vi "FPGA Target 2.vi"() -> ()   [LabVIEW 2015]
uses:
  <vilib>/Platform/TimedLoop/XDataNode/wakeup.ctl
  <vilib>/Platform/TimedLoop/XDataNode/XDNodeRunTimeDep.lvlib
  <vilib>/Platform/TimedLoop/XDataNode/nitl_modes.ctl
  <vilib>/Platform/TimedLoop/XDataNode/timing_clust.ctl
  <vilib>/Platform/TimedLoop/XDataNode/XDataNode.xnode
  <vilib>/NI/Engine Simulation Toolkit (EST)/APU/APU.lvlib
  <vilib>/rvi/DataTransferAndStorage/Container/XNode/niFpgaContainer.xnode
  <vilib>/rvi/interface/RandomDataEmulation/nirviRandomDataFpgaReadWriteTemplate.vi
  <vilib>/NI/Engine Simulation Toolkit (EST)/Digital Pattern Generation/Digital Pattern Generation.lvlib
  <vilib>/NI/Engine Simulation Toolkit (EST)/Directional Speed/Directional Speed.lvlib
  <vilib>/NI/Engine Simulation Toolkit (EST)/Analog Replay/Analog Replay.lvlib
  <vilib>/NI/FPGA Addon IP/Speciality IO/Speciality FPGA IO.lvlib
  <vilib>/NI/Engine Simulation Toolkit (EST)/Knock Sensor/Knock Sensor.lvlib
  <vilib>/NI/Engine Simulation Toolkit (EST)/ECU Event/Timing/ECU Event Timing.lvlib
  <vilib>/NI/Engine Simulation Toolkit (EST)/ECU Event/Timing/Measure Events (Non-40MHz).vi
  <vilib>/NI/Engine Simulation Toolkit (EST)/ECU Event/Timing/Capture Settings.ctl
  <vilib>/NI/Engine Simulation Toolkit (EST)/APU/Shared Settings.ctl
  <vilib>/NI/Engine Simulation Toolkit (EST)/Version Token.ctl
  <vilib>/NI/Engine Simulation Toolkit (EST)/Engine Simulation Toolkit.lvlib
  <vilib>/NI/Engine Simulation Toolkit (EST)/APU/Settings.ctl
  <vilib>/NI/Engine Simulation Toolkit (EST)/APU/Input.ctl
  <vilib>/NI/Engine Simulation Toolkit (EST)/APU/Output.ctl
  <vilib>/NI/Engine Simulation Toolkit (EST)/Digital Pattern Generation/Load Input.ctl
  <vilib>/NI/Engine Simulation Toolkit (EST)/Directional Speed/Load Input.ctl
  <vilib>/NI/Engine Simulation Toolkit (EST)/Analog Replay/Load Input.ctl
  <vilib>/NI/FPGA Addon IP/Speciality IO/Types/PWM.Measure.Analog.Settings.ctl
  <vilib>/NI/FPGA Addon IP/Speciality IO/Types/PWM.Measure.Analog.Measurement.ctl
  <vilib>/NI/Engine Simulation Toolkit (EST)/Knock Sensor/Cylinder Settings.ctl
  <vilib>/NI/Engine Simulation Toolkit (EST)/Knock Sensor/Cylinder Input.ctl
  <vilib>/NI/Engine Simulation Toolkit (EST)/Knock Sensor/Generate Settings.ctl
  <vilib>/NI/Engine Simulation Toolkit (EST)/Knock Sensor/Generate Input.ctl
  <vilib>/NI/Engine Simulation Toolkit (EST)/Analog Replay/Input.ctl
  <vilib>/NI/Engine Simulation Toolkit (EST)/Analog Replay/Settings.ctl
  <vilib>/NI/FPGA Addon IP/Speciality IO/Types/Sine.Generate.Settings.ctl
  <vilib>/NI/FPGA Addon IP/Speciality IO/Types/PWM.Generate.Digital.Settings.ctl
  <vilib>/NI/Engine Simulation Toolkit (EST)/Digital Pattern Generation/Input.ctl
  <vilib>/NI/Engine Simulation Toolkit (EST)/Digital Pattern Generation/Settings.ctl
  <vilib>/NI/Engine Simulation Toolkit (EST)/Directional Speed/Input.ctl
  <vilib>/NI/Engine Simulation Toolkit (EST)/Directional Speed/Settings.ctl
  <vilib>/NI/FPGA Addon IP/Speciality IO/Types/WSS.Generate.Digital.Settings.ctl
  <vilib>/NI/FPGA Addon IP/Speciality IO/Types/PWM.Measure.Digital.Settings.ctl
  <vilib>/NI/FPGA Addon IP/Speciality IO/Types/PWM.Measure.Digital.Measurement.ctl
  <vilib>/NI/Engine Simulation Toolkit (EST)/ECU Event/Timing/Measure Settings.ctl
  <vilib>/NI/Engine Simulation Toolkit (EST)/ECU Event/Timing/Measure Output.ctl
  <vilib>/NI/Engine Simulation Toolkit (EST)/ECU Event/Timing/Capture Output.ctl
panel:
  out "capture.Cyl Inj 3.Event 4":T1
  out "capture.Cyl Inj 3.Event 3":T1
  out "capture.Cyl Inj 3.Event 2":T1
  out "capture.Cyl Inj 3.Event 1":T1
  out "status.Cyl Inj 3":T2
  in  "settings.Cyl Inj 3":T3
  out "capture.Cyl Inj 2.Event 4":T1
  out "capture.Cyl Inj 2.Event 3":T1
  out "capture.Cyl Inj 2.Event 2":T1
  out "capture.Cyl Inj 2.Event 1":T1
  out "status.Cyl Inj 2":T2
  in  "settings.Cyl Inj 2":T3
  out "capture.Cyl Inj 1.Event 4":T1
  out "capture.Cyl Inj 1.Event 3":T1
  out "capture.Cyl Inj 1.Event 2":T1
  out "capture.Cyl Inj 1.Event 1":T1
  out "status.Cyl Inj 1":T2
  in  "settings.Cyl Inj 1":T3
  out "PWM IN 2.Measure":T4
  in  "PWM IN 2.Settings":T5={"ACTIVE EDGE"=TRUE, "TIMEOUT"=40000000}
  out "PWM IN 1.Measure":T4
  in  "PWM IN 1.Settings":T5={"ACTIVE EDGE"=TRUE, "TIMEOUT"=40000000}
  out "Key State":bool
  out "Switch State":bool
  out "Relay State":bool
  out "Connector0 DIO Bank2.Monitor":bool[](array[boolean])
  out "Connector0 DIO Bank1.Monitor":bool[](array[boolean])
  in  "Read Passenger WS.Settings":T6={"ACTIVE EDGE"=TRUE, "ACTIVE TICKS"=0, "INACTIVE TICKS"=0, "DATA"=0, "SENSOR TYPE"=0}
  in  "Rear Driver WS.Settings":T6={"ACTIVE EDGE"=TRUE, "ACTIVE TICKS"=0, "INACTIVE TICKS"=0, "DATA"=0, "SENSOR TYPE"=0}
  in  "Front Passenger WS.Settings":T6={"ACTIVE EDGE"=TRUE, "ACTIVE TICKS"=0, "INACTIVE TICKS"=0, "DATA"=0, "SENSOR TYPE"=0}
  in  "Front Driver WS.Settings":T6={"ACTIVE EDGE"=TRUE, "ACTIVE TICKS"=0, "INACTIVE TICKS"=0, "DATA"=0, "SENSOR TYPE"=0}
  out "Connector0 DIO Bank0.Monitor":bool[](array[boolean])
  in  "input.Crank":T7
  in  "settings.Crank":T8
  in  "input.Crank_Temp":T9
  in  "settings.Crank_Temp":T10
  in  "Switch":bool
  in  "Key":bool
  in  "input.Exhaust CAM 1":T9
  in  "settings.Exhaust CAM 1":T10
  in  "input.Intake CAM 1":T9
  in  "settings.Intake CAM 1":T10
  in  "PWM Out 2.Settings":T11={"ACTIVE EDGE"=TRUE, "ACTIVE TICKS"=0, "INACTIVE TICKS"=0}
  in  "PWM Out 1.Settings":T11={"ACTIVE EDGE"=TRUE, "ACTIVE TICKS"=0, "INACTIVE TICKS"=0}
  out "Connector1 AO Bank0.Monitor":fxp<+/-,32,8>[](array[numeric])
  in  "Simple Knock 2.Settings":T12={"AMP"=0.0, "OFFSET"=0.0, "PERIODS/TICKS"=2.4999957531690598e-05}
  in  "Simple Knock 1.Settings":T12={"AMP"=0.0, "OFFSET"=0.0, "PERIODS/TICKS"=2.4999957531690598e-05}
  in  "input.VR Sensor2":T13
  in  "settings.VR Sensor2":T14
  in  "input.VR Sensor1":T13
  in  "settings.VR Sensor1":T14
  in  "Power Supply Setpoint":fxp<+/-,32,8> format="%#_27g"
  in  "Dyno Setpoint":fxp<+/-,32,8> format="%#_27g"
  in  "input.Knock2":T15
  in  "settings.Knock2":T16
  in  "input.Knock2.Cylinder 7":T17={"probability compare"=65535, "high freq scaler"=0.0, "trigger position"=0}
  in  "settings.Knock2.Cylinder 7":T18
  in  "input.Knock2.Cylinder 6":T17={"probability compare"=65535, "high freq scaler"=0.0, "trigger position"=0}
  in  "settings.Knock2.Cylinder 6":T18
  in  "input.Knock2.Cylinder 5":T17={"probability compare"=65535, "high freq scaler"=0.0, "trigger position"=0}
  in  "settings.Knock2.Cylinder 5":T18
  in  "input.Knock2.Cylinder 4":T17={"probability compare"=65535, "high freq scaler"=0.0, "trigger position"=0}
  in  "settings.Knock2.Cylinder 4":T18
  in  "input.Knock2.Cylinder 3":T17={"probability compare"=65535, "high freq scaler"=0.0, "trigger position"=0}
  in  "settings.Knock2.Cylinder 3":T18
  in  "input.Knock2.Cylinder 2":T17={"probability compare"=65535, "high freq scaler"=0.0, "trigger position"=0}
  in  "settings.Knock2.Cylinder 2":T18
  in  "input.Knock2.Cylinder 1":T17={"probability compare"=65535, "high freq scaler"=0.0, "trigger position"=0}
  in  "settings.Knock2.Cylinder 1":T18
  in  "input.Knock1":T15
  in  "settings.Knock1":T16
  in  "input.Knock1.Cylinder 6":T17={"probability compare"=65535, "high freq scaler"=0.0, "trigger position"=0}
  in  "settings.Knock1.Cylinder 6":T18
  in  "input.Knock1.Cylinder 5":T17={"probability compare"=65535, "high freq scaler"=0.0, "trigger position"=0}
  in  "settings.Knock1.Cylinder 5":T18
  in  "input.Knock1.Cylinder 4":T17={"probability compare"=65535, "high freq scaler"=0.0, "trigger position"=0}
  in  "settings.Knock1.Cylinder 4":T18
  in  "input.Knock1.Cylinder 3":T17={"probability compare"=65535, "high freq scaler"=0.0, "trigger position"=0}
  in  "settings.Knock1.Cylinder 3":T18
  in  "input.Knock1.Cylinder 2":T17={"probability compare"=65535, "high freq scaler"=0.0, "trigger position"=0}
  in  "settings.Knock1.Cylinder 2":T18
  in  "input.Knock1.Cylinder 1":T17={"probability compare"=65535, "high freq scaler"=0.0, "trigger position"=0}
  in  "settings.Knock1.Cylinder 1":T18
  out "Temp2":fxp<+/-,32,8> format="%#_27g"
  out "Temp1":fxp<+/-,32,8> format="%#_27g"
  out "Pressure4":fxp<+/-,32,8> format="%#_27g"
  out "Pressure3":fxp<+/-,32,8> format="%#_27g"
  out "Injector4.Measure":T19
  in  "Injector4.Settings":T20={"ACTIVE EDGE"=TRUE, "TIMEOUT"=40000000, "THRESHOLD"=50.0}
  out "Injector3.Measure":T19
  in  "Injector3.Settings":T20={"ACTIVE EDGE"=TRUE, "TIMEOUT"=40000000, "THRESHOLD"=50.0}
  out "Pressure2":fxp<+/-,32,8> format="%#_27g"
  out "Pressure1":fxp<+/-,32,8> format="%#_27g"
  out "Connector1 AI Bank0.Monitor":fxp<+/-,27,5>[](array[numeric])
  in  "load input.VR Sensor2":T21={"Data"=[0, 0, 0, 0, 0, 0, 0, 0, 0, 0, 0, 0, 0, 0, 0, 0], "LoadOffset"=0, "Done"=FALSE}
  in  "load input.VR Sensor1":T21={"Data"=[0, 0, 0, 0, 0, 0, 0, 0, 0, 0, 0, 0, 0, 0, 0, 0], "LoadOffset"=0, "Done"=FALSE}
  in  "load input.Crank":T22
  in  "load input.Crank_Temp":T23
  in  "load input.Exhaust CAM 1":T23
  in  "load input.Intake CAM 1":T23
  in  "Analog Input Loop Timer (uSec)":u32
  out "output.apu 1":T24 caption="output"
  in  "input.apu 1":T25={"desired speed"=0.0, "reset"=TRUE} caption="input"
  in  "settings.apu 1":T26 caption="settings"
  in  "est.version":T27
  in  "shared settings.apu 1":T28 {"start" format="%#.15g"}
  in  "go.apu 1":bool
  in  "Digital Loop Timer (uSec)":u32
  in  "Analog Output Loop Timer (uSec)":u32
  in  "DMA.Enable":bool
  in  "DMA.MinimumSamples":u32 caption="DMA Loop Timer (uSec)"
  out "DMA.Timeout":bool
  in  "DMA.Timeout.Reset":bool
  in  "DMA Loop Timer (uSec)":u32
types:
  T1 = typedef "Engine Simulation Toolkit.lvlib/ECU Event Timing.lvlib/Capture Output.ctl" = cluster{"Start":u16, "End":u16, "Duration (tics)":fxp<+,18,18>, "Event present":bool}
  T2 = typedef "Engine Simulation Toolkit.lvlib/ECU Event Timing.lvlib/Measure Output.ctl" = cluster{"stuck active":bool, "window all active":bool, "window orphan start":bool, "window orphan end":bool}
  T3 = typedef "Engine Simulation Toolkit.lvlib/ECU Event Timing.lvlib/Measure Settings.ctl" = cluster{"max":u16, "min":u16, "active high":bool, "wrap":bool}
  T4 = typedef "Speciality FPGA IO.lvlib/PWM.Measure.Digital.Measurement.ctl" = cluster{"ACTIVE TICKS":u32, "INACTIVE TICKS":u32, "ACQ TICKS":u32}
  T5 = typedef "Speciality FPGA IO.lvlib/PWM.Measure.Digital.Settings.ctl" = cluster{"ACTIVE EDGE":bool, "TIMEOUT":u32}
  T6 = typedef "Speciality FPGA IO.lvlib/WSS.Generate.Digital.Settings.ctl" = cluster{"ACTIVE EDGE":bool, "ACTIVE TICKS":u32, "INACTIVE TICKS":u32, "DATA":u8, "SENSOR TYPE":u8}
  T7 = typedef "Engine Simulation Toolkit.lvlib/Directional Speed.lvlib/Settings.ctl" = cluster{"Upper Value":u16, "Lower Value":u16, "Upper Index":fxp<+,10,10>, "Lower Index":fxp<+,10,10>, "Enabled":bool}
  T8 = typedef "Engine Simulation Toolkit.lvlib/Directional Speed.lvlib/Input.ctl" = cluster{"td (tics)":u16, "tf (tics)":u16, "tr (tics)":u16}
  T9 = typedef "Engine Simulation Toolkit.lvlib/Digital Pattern Generation.lvlib/Settings.ctl" = cluster{"edge 1":u16, "edge 2":u16, "cycle angle":bool, "enabled":bool, "first falling":bool, "fault":bool, "fault wrap":bool, "fault value":bool, "fault count":fxp<+,4,4>, "use fault count":bool}
  T10 = typedef "Engine Simulation Toolkit.lvlib/Digital Pattern Generation.lvlib/Input.ctl" = cluster{"Offset":i16}
  T11 = typedef "Speciality FPGA IO.lvlib/PWM.Generate.Digital.Settings.ctl" = cluster{"ACTIVE EDGE":bool, "ACTIVE TICKS":u32, "INACTIVE TICKS":u32}
  T12 = typedef "Speciality FPGA IO.lvlib/Sine.Generate.Settings.ctl" = cluster{"AMP":fxp<+/-,32,8>, "OFFSET":fxp<+/-,32,8>, "PERIODS/TICKS":fxp<+,32,0>}
  T13 = typedef "Engine Simulation Toolkit.lvlib/Analog Replay.lvlib/Settings.ctl" = cluster{"ReverseNegate":bool, "CycleAngle":bool, "SpeedThreshold":fxp<+/-,23,2>, "AOBelowThreshold":i16}
  T14 = typedef "Engine Simulation Toolkit.lvlib/Analog Replay.lvlib/Input.ctl" = cluster{"Offset":i16, "VScaleSlope":fxp<+,18,6>, "VScaleIntercept":fxp<+/-,18,3>}
  T15 = typedef "Engine Simulation Toolkit.lvlib/Knock Sensor.lvlib/Generate Input.ctl" = cluster{"low freq scaler":fxp<+,10,0>}
  T16 = typedef "Engine Simulation Toolkit.lvlib/Knock Sensor.lvlib/Generate Settings.ctl" = cluster{"low freq (periods/tick)":fxp<+,32,0>, "high freq (periods/tick)":fxp<+,32,0>, "duration (1.25MHz tics)":fxp<+,18,18>, "low freq speed slope":fxp<+,16,-3>, "low freq speed intercept":fxp<+,10,-10>, "low freq by speed":bool}
  T17 = typedef "Engine Simulation Toolkit.lvlib/Knock Sensor.lvlib/Cylinder Input.ctl" = cluster{"probability compare":u16, "high freq scaler":fxp<+,10,0>, "trigger position":u16}
  T18 = typedef "Engine Simulation Toolkit.lvlib/Knock Sensor.lvlib/Cylinder Settings.ctl" = cluster{"seed":u16, "reset":bool}
  T19 = typedef "Speciality FPGA IO.lvlib/PWM.Measure.Analog.Measurement.ctl" = cluster{"ACTIVE TICKS":u32, "INACTIVE TICKS":u32, "ACQ TICKS":u32, "ACTIVE VOLTAGE":fxp<+/-,32,8>, "INACTIVE VOLTAGE":fxp<+/-,32,8>}
  T20 = typedef "Speciality FPGA IO.lvlib/PWM.Measure.Analog.Settings.ctl" = cluster{"ACTIVE EDGE":bool, "TIMEOUT":u32, "THRESHOLD":fxp<+/-,32,8>}
  T21 = typedef "Engine Simulation Toolkit.lvlib/Analog Replay.lvlib/Load Input.ctl" = cluster{"Data":i16[], "LoadOffset":u16, "Done":bool}
  T22 = typedef "Engine Simulation Toolkit.lvlib/Directional Speed.lvlib/Load Input.ctl" = cluster{"address":fxp<+,10,10>, "done":bool, "angle":u16}
  T23 = typedef "Engine Simulation Toolkit.lvlib/Digital Pattern Generation.lvlib/Load Input.ctl" = cluster{"address":fxp<+,11,11>, "done":bool, "angle":u16}
  T24 = typedef "Engine Simulation Toolkit.lvlib/APU.lvlib/Output.ctl" = cluster{"crank":u16, "cycle":u16, "actual speed":fxp<+/-,23,2>}
  T25 = typedef "Engine Simulation Toolkit.lvlib/APU.lvlib/Input.ctl" = cluster{"desired speed":fxp<+/-,23,2>, "reset":bool}
  T26 = typedef "Engine Simulation Toolkit.lvlib/APU.lvlib/Settings.ctl" = cluster{"acceleration":fxp<+,18,-20>, "enable accel":bool}
  T27 = typedef "Engine Simulation Toolkit.lvlib/Version Token.ctl" = cluster{"1.3.0":bool}
  T28 = typedef "Engine Simulation Toolkit.lvlib/APU.lvlib/Shared Settings.ctl" = cluster{"start":fxp<+,17,17>, "stuck limit":fxp<+,18,18>}
  T29 = typedef "XDNodeRunTimeDep.lvlib/timing_clust.ctl" = cluster{"Expected End [f-1]":u64, "Actual End [f-1]":u64, "Finished Late? [f-1]":bool, "Expected End [i-1]":u64, "Actual End [i-1]":u64, "Finished Late? [i-1]":bool, "Expected Start [i]":u64, "Actual Start [i]":u64, "Expected Start [f]":u64, "Actual Start [f]":u64, "Source Name":string, "Structure Name":string, "Period":i64, "Deadline":i64, "Offset":i64, "Start":i64, "Priority":i32, "Timeout":i32, "Mode":T30, "Wakeup Reason":T31, "Error":errorcluster, "Source Type":string, "Secondary Source Type":string, "Global End Time":u64, "Global Start Time":u64, "Frame Duration":u64, "Iteration Duration":u64, "Assigned CPU":i32, "I/O Scan Engine Mode":u32}
  T30 = typedef "XDNodeRunTimeDep.lvlib/nitl_modes.ctl" = enum32{"No Change", "Process missed periods, maintain original phase", "Discard missed periods, maintain original phase", "Process missed periods, ignore original phase", "Discard missed periods, ignore original phase"}
  T31 = typedef "XDNodeRunTimeDep.lvlib/wakeup.ctl" = enum32{"Normal", "Aborted", "Asynchronous wakeup", "Timing source error", "Timed loop error", "Timeout"}
  T32 = typedef "Engine Simulation Toolkit.lvlib/ECU Event Timing.lvlib/Capture Settings.ctl" = u8
  T33 = cluster{"DI 0":refnum<k21>, "DI 1":refnum<k21>, "DI 2":refnum<k21>, "DI 3":refnum<k21>, "DI 4":refnum<k21>, "DI 5":refnum<k21>, "DI 6":refnum<k21>, "DI 7":refnum<k21>}
  T34 = cluster{"DO 0":refnum<k21>, "DO 1":refnum<k21>, "DO 2":refnum<k21>, "DO 3":refnum<k21>, "DO 4":refnum<k21>, "DO 5":refnum<k21>, "DO 6":refnum<k21>, "DO 7":refnum<k21>}
  T35 = cluster{"AO 0":refnum<k21>, "AO 1":refnum<k21>, "AO 2":refnum<k21>, "AO 3":refnum<k21>, "AO 4":refnum<k21>, "AO 5":refnum<k21>, "AO 6":refnum<k21>, "AO 7":refnum<k21>}
  T36 = cluster{"AI 0":refnum<k21>, "AI 1":refnum<k21>, "AI 2":refnum<k21>, "AI 3":refnum<k21>, "AI 4":refnum<k21>, "AI 5":refnum<k21>, "AI 6":refnum<k21>, "AI 7":refnum<k21>}
  T37 = typedef "Engine Simulation Toolkit.lvlib/APU.lvlib/Register Bus.ctl" = cluster{"Speed":refnum<k21>, "Crank Angle":refnum<k21>, "Cycle Angle":refnum<k21>, "Crank Count":refnum<k21>, "Cycle Count":refnum<k21>, "1.25 MHz Counter":refnum<k21>, "Crank Rollover":refnum<k21>, "Cycle Rollover":refnum<k21>, "shared settings":T28}
  T38 = typedef "Engine Simulation Toolkit.lvlib/Digital Pattern Generation.lvlib/Load Data.ctl" = cluster{"max address":fxp<+,11,11>, "memory":refnum<k21>}
  T39 = typedef "Engine Simulation Toolkit.lvlib/Directional Speed.lvlib/Load Data.ctl" = cluster{"max address":fxp<+,10,10>, "Memory":refnum<k21>}
  T40 = typedef "Engine Simulation Toolkit.lvlib/Knock Sensor.lvlib/Triggered Cylinder Data.ctl" = cluster{"trigger knock":bool, "high freq scaler":fxp<+,10,0>}
  T41 = typedef "Engine Simulation Toolkit.lvlib/ECU Event Timing.lvlib/Measured Data.ctl" = cluster{"start":u16, "end":u16, "duration (tics)":fxp<+,18,18>, "window end":bool, "window begin":bool, "pulse end":bool, "pulse #":u8}
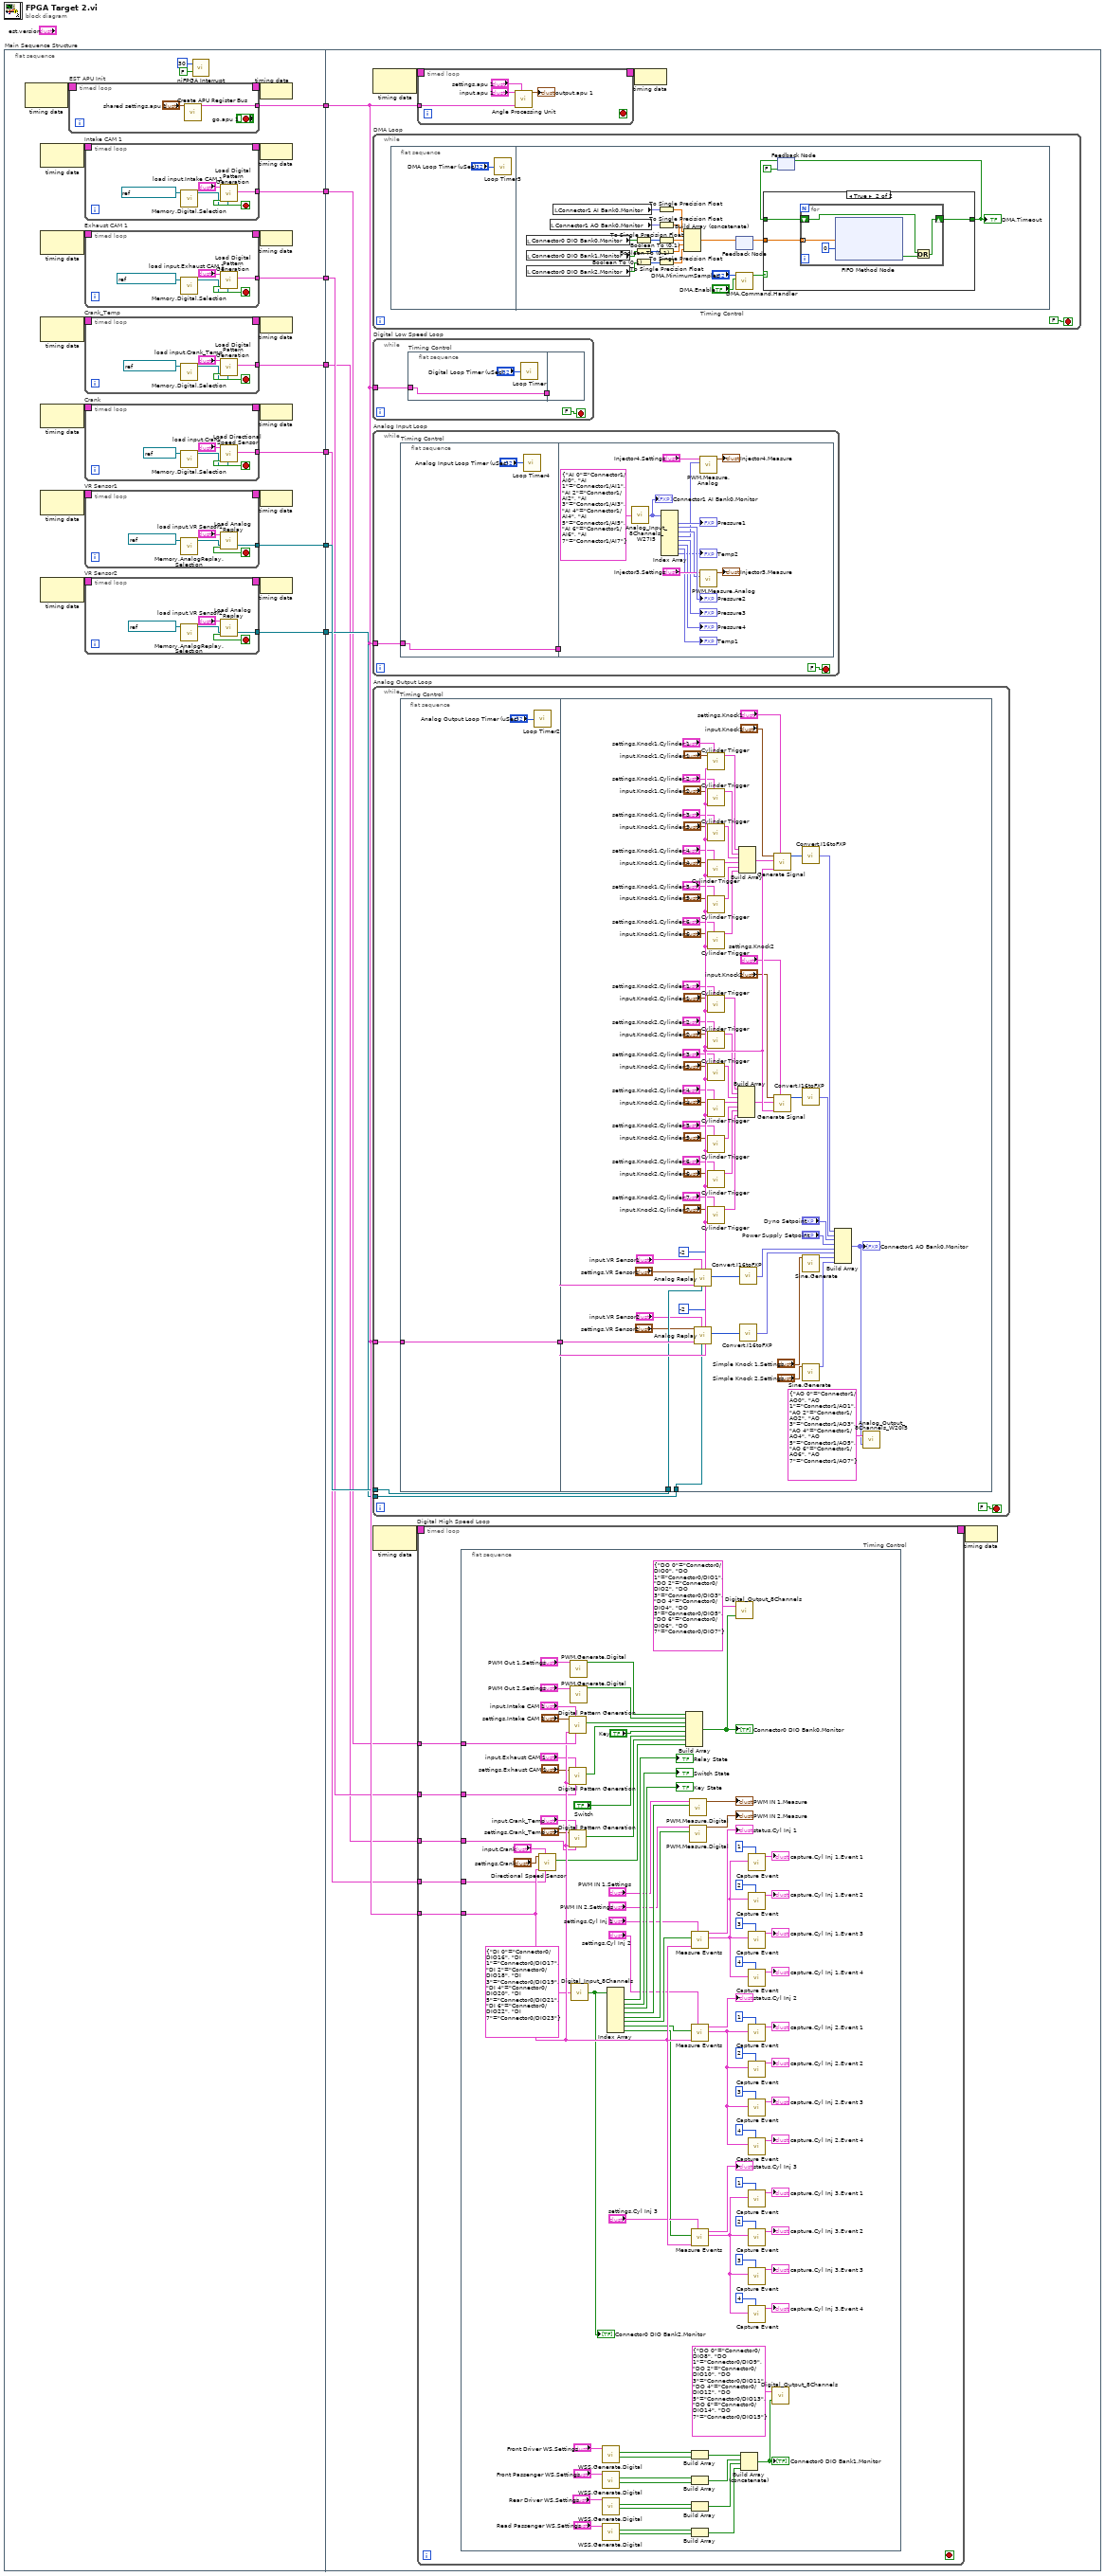
[diagram p0: block diagram]
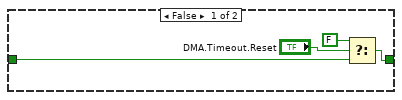
[diagram p2: hidden frame]
diagram:
  n1 = flat-sequence "Main Sequence Structure" {
    tunnel: [w26] -> w7
    tunnel: [w13] -> w6
    tunnel: [w12] -> w5
    tunnel: [w11] -> w4
    tunnel: [w10] -> w3
    tunnel: [w9] -> w2
    tunnel: [w8] -> w1
    tunnel: w7 -> [w96]
    tunnel: w6 -> [w95]
    tunnel: w5 -> [w94]
    tunnel: w4 -> [w93]
    tunnel: w3 -> [w92]
    tunnel: w2 -> [w91]
    tunnel: w1 -> [w90]
    frame #0 {
      n2 = node-c288() -> (w28:T29)  [unwired: 1 in]
      n3 = node-c288() -> (w25:T29)  [unwired: 1 in]
      n4 = node-c288() -> (w23:T29)  [unwired: 1 in]
      n5 = node-c288() -> (w21:T29)  [unwired: 1 in]
      n6 = node-c288() -> (w19:T29)  [unwired: 1 in]
      n7 = node-c288() -> (w17:T29)  [unwired: 1 in]
      n8 = node-c288() -> (w15:T29)  [unwired: 1 in]
      n9 = timed-loop "EST APU Init" {
        timing: w28 -> [_]
        timing-out: [_] -> w27
        tunnel: [w83] -> w26
        stop <- "go.apu 1" stop-if-true
        n10 = call <vilib>:"Create APU Register Bus.vi"("shared settings.<user name>"="shared settings.apu 1") -> ("register bus"=w83:T37)  [unwired: 10 in]
      }
      n11 = timed-loop "Intake CAM 1" {
        timing: w25 -> [_]
        timing-out: [_] -> w24
        tunnel: [w74] -> w11
        stop <- w77 stop-if-true
        n12 = call "Memory.Digital.Selection.vi"("memory"=refnum<k21> "Intake CAM 1") -> ("memory"=w75:refnum<k21>)  [unwired: 10 in]
        n13 = call <vilib>:"Load Digital Pattern Generation.vi"("memory"=w75, "load input.<user name>"="load input.Intake CAM 1") -> ("done"=w77:bool, "load data"=w74:T38)  [unwired: 8 in]
      }
      n14 = timed-loop "Exhaust CAM 1" {
        timing: w23 -> [_]
        timing-out: [_] -> w22
        tunnel: [w65] -> w10
        stop <- w68 stop-if-true
        n15 = call "Memory.Digital.Selection.vi"("memory"=refnum<k21> "Exhaust CAM 1") -> ("memory"=w66:refnum<k21>)  [unwired: 10 in]
        n16 = call <vilib>:"Load Digital Pattern Generation.vi"("memory"=w66, "load input.<user name>"="load input.Exhaust CAM 1") -> ("done"=w68:bool, "load data"=w65:T38)  [unwired: 8 in]
      }
      n17 = timed-loop "Crank_Temp" {
        timing: w21 -> [_]
        timing-out: [_] -> w20
        tunnel: [w56] -> w9
        stop <- w59 stop-if-true
        n18 = call "Memory.Digital.Selection.vi"("memory"=refnum<k21> "Crank_Temp") -> ("memory"=w57:refnum<k21>)  [unwired: 10 in]
        n19 = call <vilib>:"Load Digital Pattern Generation.vi"("memory"=w57, "load input.<user name>"="load input.Crank_Temp") -> ("done"=w59:bool, "load data"=w56:T38)  [unwired: 8 in]
      }
      n20 = timed-loop "Crank" {
        timing: w19 -> [_]
        timing-out: [_] -> w18
        tunnel: [w47] -> w8
        stop <- w50 stop-if-true
        n21 = call "Memory.Digital.Selection.vi"("memory"=refnum<k21> "Crank") -> ("memory"=w48:refnum<k21>)  [unwired: 10 in]
        n22 = call <vilib>:"Load Directional Speed Sensor.vi"("Memory In"=w48, "load input.<user name>"="load input.Crank") -> ("done"=w50:bool, "load data"=w47:T39)  [unwired: 8 in]
      }
      n23 = timed-loop "VR Sensor1" {
        timing: w17 -> [_]
        timing-out: [_] -> w16
        tunnel: [w39] -> w13
        stop <- w41 stop-if-true
        n24 = call "Memory.AnalogReplay.Selection.vi"("memory"=refnum<k21> "VR Sensor1") -> ("memory"=w39:refnum<k21>)  [unwired: 10 in]
        n25 = call <vilib>:"Load Analog Replay.vi"("memory"=w39, "load input.<user name>"="load input.VR Sensor1") -> ("done"=w41:bool)  [unwired: 9 in]
      }
      n26 = timed-loop "VR Sensor2" {
        timing: w15 -> [_]
        timing-out: [_] -> w14
        tunnel: [w31] -> w12
        stop <- w33 stop-if-true
        n27 = call "Memory.AnalogReplay.Selection.vi"("memory"=refnum<k21> "VR Sensor2") -> ("memory"=w31:refnum<k21>)  [unwired: 10 in]
        n28 = call <vilib>:"Load Analog Replay.vi"("memory"=w31, "load input.<user name>"="load input.VR Sensor2") -> ("done"=w33:bool)  [unwired: 9 in]
      }
      n29 = call <vilib>:"niFPGA Interrupt.vi"("Wait Until Cleared (F)"=FALSE, "IRQ Number (0)"=u8 30) -> ()  [unwired: 1 in]
      n30 = node-c288(w27) -> ()
      n31 = node-c288(w24) -> ()
      n32 = node-c288(w22) -> ()
      n33 = node-c288(w20) -> ()
      n34 = node-c288(w18) -> ()
      n35 = node-c288(w16) -> ()
      n36 = node-c288(w14) -> ()
    }
    frame #1 {
      # "FPGA Addon Code"
      n37 = node-c288 ("Input Node")() -> (w98:T29)  [unwired: 1 in]
      n38 = while "DMA Loop" {
        stop <- FALSE stop-if-true
        n39 = flat-sequence "Timing Control" {
          frame #0 {
            n40 = call "Loop Timer3"("Count(uSec)"="DMA Loop Timer (uSec)") -> ()  [unwired: 1 out]
          }
          frame #1 {
            n41 = local read "Connector0 DIO Bank0.Monitor"() -> (w220:bool[])
            n42 = local read "Connector0 DIO Bank1.Monitor"() -> (w218:bool[])
            n43 = local read "Connector0 DIO Bank2.Monitor"() -> (w216:bool[])
            n44 = local read "Connector1 AO Bank0.Monitor"() -> (w221:fxp<+/-,32,8>[])
            n45 = local read "Connector1 AI Bank0.Monitor"() -> (w222:fxp<+/-,27,5>[])
            n46 = Boolean To (0,1)(Boolean=w220) -> (0, 1=w219:i16[])
            n47 = Boolean To (0,1)(Boolean=w218) -> (0, 1=w217:i16[])
            n48 = Boolean To (0,1)(Boolean=w216) -> (0, 1=w215:i16[])
            n49 = To Single Precision Float(number=w222) -> (single precision float=w214:sgl[])
            n50 = To Single Precision Float(number=w221) -> (single precision float=w213:sgl[])
            n51 = To Single Precision Float(number=w219) -> (single precision float=w212:sgl[])
            n52 = To Single Precision Float(number=w217) -> (single precision float=w211:sgl[])
            n53 = To Single Precision Float(number=w215) -> (single precision float=w210:sgl[])
            n54 = Build Array (concatenate) "Build Array"(w214, w213, w212, w211, w210) -> (w228:sgl[])
            n55 = feedback #1() -> (w227:sgl[])  [unwired: 1 in]
            n56 = feedback-in #1(w228) -> ()
            n57 = call "DMA.Command.Handler.vi"("DMA.Enable"="DMA.Enable", "DMA.MinimumSamples"="DMA.MinimumSamples") -> ("Transfer"=w224:bool)  [unwired: 9 in]
            n58 = feedback #2(FALSE ("t")) -> (w223:bool)
            n59 = case shown="True" w224 {
              tunnel: w227 -> [_ w237]
              tunnel: w223 -> [w232 w236]
              tunnel: [w231 w235] -> w226
              frame False {
                n60 = Select(t=FALSE, s="DMA.Timeout.Reset", f=w232) -> (s? t:f=w231:bool)
              }
              frame True {
                n61 = for {
                  shift-right: [w240] -> w235
                  shift-left: w236 -> [w239]
                  tunnel: w237 -> [w238] mode=indexing
                  n62 = xnode ("FIFO Method Node")("Element"=w238, "Timeout"=0) -> ("Timed Out?"=w241:bool)  [unwired: 1 in, 1 out]
                  n63 = Or(x=w239, y=w241) -> (x .or. y?=w240:bool)
                }
              }
            }
            "DMA.Timeout" <- w226
            n64 = feedback-in #2(w226) -> ()
          }
        }
      }
      n65 = while "Digital Low Speed Loop" {
        tunnel: w96 -> [w340]
        stop <- FALSE stop-if-true
        n66 = flat-sequence "Timing Control" {
          tunnel: w340 -> [w342]
          tunnel: [w342] -> w339
          tunnel: w339 -> [_]
          frame #0 {
            n67 = call "Loop Timer"("Count(uSec)"="Digital Loop Timer (uSec)") -> ()  [unwired: 1 out]
          }
          frame #1 {
          }
        }
      }
      n68 = while "Analog Input Loop" {
        tunnel: w96 -> [w321]
        stop <- FALSE stop-if-true
        n69 = flat-sequence "Timing Control" {
          tunnel: w321 -> [w323]
          tunnel: [w323] -> w320
          tunnel: w320 -> [_]
          frame #0 {
            n70 = call "Loop Timer4"("Count(uSec)"="Analog Input Loop Timer (uSec)") -> ()  [unwired: 1 out]
          }
          frame #1 {
            n71 = call "Analog_Input_8Channels_W27I5.vi"("IO"=T36 {"AI 0"="Connector1/AI0", "AI 1"="Connector1/AI1", "AI 2"="Connector1/AI2", "AI 3"="Connector1/AI3", "AI 4"="Connector1/AI4", "AI 5"="Connector1/AI5", "AI 6"="Connector1/AI6", "AI 7"="Connector1/AI7"}) -> ("Values"=w337:fxp<+/-,27,5>[])
            "Connector1 AI Bank0.Monitor" <- w337
            n72 = Index Array(array=w337) -> (element #1=→"Pressure1":fxp<+/-,27,5>, element #2=→"Pressure2":fxp<+/-,27,5>, element #3=w333:fxp<+/-,27,5>, element #4=w330:fxp<+/-,27,5>, element #5=→"Pressure3":fxp<+/-,27,5>, element #6=→"Pressure4":fxp<+/-,27,5>, element #7=→"Temp1":fxp<+/-,27,5>, element #8=→"Temp2":fxp<+/-,27,5>)  [unwired: 8 in]
            n73 = call <vilib>:"PWM.Measure.Analog.vi"("PWM"=w330, "Settings"="Injector4.Settings") -> ("Measurement"=→"Injector4.Measure":T19)  [unwired: 8 in, 1 out]
            n74 = call <vilib>:"PWM.Measure.Analog.vi"("PWM"=w333, "Settings"="Injector3.Settings") -> ("Measurement"=→"Injector3.Measure":T19)  [unwired: 8 in, 1 out]
          }
        }
      }
      n75 = while "Analog Output Loop" {
        tunnel: w96 -> [w246]
        tunnel: w95 -> [w244]
        tunnel: w94 -> [w243]
        stop <- FALSE stop-if-true
        n76 = flat-sequence "Timing Control" {
          tunnel: w246 -> [w248]
          tunnel: [w248] -> w245
          tunnel: w245 -> [w317]
          tunnel: w244 -> [w268]
          tunnel: w243 -> [w263]
          frame #0 {
            n77 = call "Loop Timer2"("Count(uSec)"="Analog Output Loop Timer (uSec)") -> ()  [unwired: 1 out]
          }
          frame #1 {
            n78 = call <vilib>:"Analog Replay.vi"("shift"=i8 -2, "memory"=w268, "settings.<user name>"="input.VR Sensor1", "register bus"=w317, "input.<user name>"="settings.VR Sensor1") -> ("analog value"=w267:i16)  [unwired: 6 in]
            n79 = call <vilib>:"Analog Replay.vi"("shift"=i8 -2, "memory"=w263, "settings.<user name>"="input.VR Sensor2", "register bus"=w317, "input.<user name>"="settings.VR Sensor2") -> ("analog value"=w262:i16)  [unwired: 6 in]
            n80 = call <vilib>:"Cylinder Trigger.vi"("settings.<user name>"="settings.Knock1.Cylinder 1", "register bus"=w317, "input.<user name>"="input.Knock1.Cylinder 1") -> ("triggered knock data"=w316:T40)  [unwired: 8 in]
            n81 = call <vilib>:"Cylinder Trigger.vi"("settings.<user name>"="settings.Knock1.Cylinder 2", "register bus"=w317, "input.<user name>"="input.Knock1.Cylinder 2") -> ("triggered knock data"=w313:T40)  [unwired: 8 in]
            n82 = call <vilib>:"Cylinder Trigger.vi"("settings.<user name>"="settings.Knock1.Cylinder 3", "register bus"=w317, "input.<user name>"="input.Knock1.Cylinder 3") -> ("triggered knock data"=w310:T40)  [unwired: 8 in]
            n83 = call <vilib>:"Cylinder Trigger.vi"("settings.<user name>"="settings.Knock1.Cylinder 4", "register bus"=w317, "input.<user name>"="input.Knock1.Cylinder 4") -> ("triggered knock data"=w307:T40)  [unwired: 8 in]
            n84 = call <vilib>:"Cylinder Trigger.vi"("settings.<user name>"="settings.Knock1.Cylinder 5", "register bus"=w317, "input.<user name>"="input.Knock1.Cylinder 5") -> ("triggered knock data"=w304:T40)  [unwired: 8 in]
            n85 = call <vilib>:"Cylinder Trigger.vi"("settings.<user name>"="settings.Knock1.Cylinder 6", "register bus"=w317, "input.<user name>"="input.Knock1.Cylinder 6") -> ("triggered knock data"=w301:T40)  [unwired: 8 in]
            n86 = call <vilib>:"Cylinder Trigger.vi"("settings.<user name>"="settings.Knock2.Cylinder 1", "register bus"=w317, "input.<user name>"="input.Knock2.Cylinder 1") -> ("triggered knock data"=w294:T40)  [unwired: 8 in]
            n87 = call <vilib>:"Cylinder Trigger.vi"("settings.<user name>"="settings.Knock2.Cylinder 2", "register bus"=w317, "input.<user name>"="input.Knock2.Cylinder 2") -> ("triggered knock data"=w291:T40)  [unwired: 8 in]
            n88 = call <vilib>:"Cylinder Trigger.vi"("settings.<user name>"="settings.Knock2.Cylinder 3", "register bus"=w317, "input.<user name>"="input.Knock2.Cylinder 3") -> ("triggered knock data"=w288:T40)  [unwired: 8 in]
            n89 = call <vilib>:"Cylinder Trigger.vi"("settings.<user name>"="settings.Knock2.Cylinder 4", "register bus"=w317, "input.<user name>"="input.Knock2.Cylinder 4") -> ("triggered knock data"=w285:T40)  [unwired: 8 in]
            n90 = call <vilib>:"Cylinder Trigger.vi"("settings.<user name>"="settings.Knock2.Cylinder 5", "register bus"=w317, "input.<user name>"="input.Knock2.Cylinder 5") -> ("triggered knock data"=w282:T40)  [unwired: 8 in]
            n91 = call <vilib>:"Cylinder Trigger.vi"("settings.<user name>"="settings.Knock2.Cylinder 6", "register bus"=w317, "input.<user name>"="input.Knock2.Cylinder 6") -> ("triggered knock data"=w279:T40)  [unwired: 8 in]
            n92 = call <vilib>:"Cylinder Trigger.vi"("settings.<user name>"="settings.Knock2.Cylinder 7", "register bus"=w317, "input.<user name>"="input.Knock2.Cylinder 7") -> ("triggered knock data"=w276:T40)  [unwired: 8 in]
            n93 = Build Array(w294, w291, w288, w285, w282, w279, w276) -> (w273:T40[])
            n94 = Build Array(w316, w313, w310, w307, w304, w301) -> (w298:T40[])
            n95 = call "Convert.I16toFXP.vi"("16bit integer"=w267) -> ("x*y"=w255:fxp<+/-,20,5>)  [unwired: 4 in]
            n96 = call "Convert.I16toFXP.vi"("16bit integer"=w262) -> ("x*y"=w254:fxp<+/-,20,5>)  [unwired: 4 in]
            n97 = call <vilib>:"Generate Signal.vi"("settings.<user name>"="settings.Knock1", "register bus"=w317, "triggered knock data"=w298, "input.<user name>"="input.Knock1") -> ("knock signal"=w297:i16)  [unwired: 7 in]
            n98 = call <vilib>:"Generate Signal.vi"("settings.<user name>"="settings.Knock2", "register bus"=w317, "triggered knock data"=w273, "input.<user name>"="input.Knock2") -> ("knock signal"=w272:i16)  [unwired: 7 in]
            n99 = call "Convert.I16toFXP.vi"("16bit integer"=w297) -> ("x*y"=w259:fxp<+/-,20,5>)  [unwired: 4 in]
            n100 = call "Convert.I16toFXP.vi"("16bit integer"=w272) -> ("x*y"=w258:fxp<+/-,20,5>)  [unwired: 4 in]
            n101 = call <vilib>:"Sine.Generate.vi"("Settings"="Simple Knock 1.Settings") -> ("Output"=w253:fxp<+/-,32,8>)  [unwired: 10 in]
            n102 = call <vilib>:"Sine.Generate.vi"("Settings"="Simple Knock 2.Settings") -> ("Output"=w252:fxp<+/-,32,8>)  [unwired: 10 in]
            n103 = Build Array(w259, w258, "Dyno Setpoint", "Power Supply Setpoint", w255, w254, w253, w252) -> (w250:fxp<+/-,32,8>[])
            "Connector1 AO Bank0.Monitor" <- w250
            n104 = call "Analog_Output_8Channels_W20I5.vi"("Values"=w250, "IO"=T35 {"AO 0"="Connector1/AO0", "AO 1"="Connector1/AO1", "AO 2"="Connector1/AO2", "AO 3"="Connector1/AO3", "AO 4"="Connector1/AO4", "AO 5"="Connector1/AO5", "AO 6"="Connector1/AO6", "AO 7"="Connector1/AO7"}) -> ()  [unwired: 1 in]
          }
        }
      }
      n105 = node-c288() -> (w100:T29)  [unwired: 1 in]
      n106 = timed-loop "Timed Loop" {
        timing: w98 -> [_]
        timing-out: [_] -> w97
        tunnel: w96 -> [w101]
        stop <- _ stop-if-true
        n107 = call <vilib>:"Angle Processing Unit.vi"("settings.<user name>"="settings.apu 1", "register bus"=w101, "input.<user name>"="input.apu 1") -> ("output.<user name>"=→"output.apu 1":T24)  [unwired: 8 in]
      }
      n108 = timed-loop "Digital High Speed Loop" {
        timing: w100 -> [_]
        timing-out: [_] -> w99
        tunnel: w96 -> [w113]
        tunnel: w93 -> [w112]
        tunnel: w92 -> [w111]
        tunnel: w91 -> [w110]
        tunnel: w90 -> [w109]
        stop <- _ stop-if-true
        n109 = flat-sequence "Timing Control" {
          tunnel: w113 -> [w198]
          tunnel: w112 -> [w199]
          tunnel: w111 -> [w195]
          tunnel: w110 -> [w192]
          tunnel: w109 -> [w189]
          frame #0 {
            n110 = call <vilib>:"Directional Speed Sensor.vi"("load data"=w189, "settings.<user name>"="input.Crank", "register bus"=w198, "input.<user name>"="settings.Crank") -> ("digial output"=w181:bool)  [unwired: 7 in]
            n111 = call <vilib>:"Digital Pattern Generation.vi"("load data"=w199, "settings.<user name>"="input.Intake CAM 1", "register bus"=w198, "input.<user name>"="settings.Intake CAM 1") -> ("digial output"=w186:bool)  [unwired: 7 in]
            n112 = call <vilib>:"Digital Pattern Generation.vi"("load data"=w195, "settings.<user name>"="input.Exhaust CAM 1", "register bus"=w198, "input.<user name>"="settings.Exhaust CAM 1") -> ("digial output"=w185:bool)  [unwired: 7 in]
            n113 = call <vilib>:"Digital Pattern Generation.vi"("load data"=w192, "settings.<user name>"="input.Crank_Temp", "register bus"=w198, "input.<user name>"="settings.Crank_Temp") -> ("digial output"=w182:bool)  [unwired: 7 in]
            n114 = call <vilib>:"PWM.Generate.Digital.vi"("Settings"="PWM Out 1.Settings") -> ("Output"=w188:bool)  [unwired: 10 in]
            n115 = call <vilib>:"PWM.Generate.Digital.vi"("Settings"="PWM Out 2.Settings") -> ("Output"=w187:bool)  [unwired: 10 in]
            n116 = call "Digital_Input_8Channels.vi"("IO"=T33 {"DI 0"="Connector0/DIO16", "DI 1"="Connector0/DIO17", "DI 2"="Connector0/DIO18", "DI 3"="Connector0/DIO19", "DI 4"="Connector0/DIO20", "DI 5"="Connector0/DIO21", "DI 6"="Connector0/DIO22", "DI 7"="Connector0/DIO23"}) -> ("States"=w159:bool[])
            "Connector0 DIO Bank2.Monitor" <- w159
            n117 = call <vilib>:"WSS.Generate.Digital.vi"("LF Wheel Speed Sensor Settings"="Front Driver WS.Settings") -> ("Bit1"=w176:bool, "Bit0"=w177:bool)  [unwired: 9 in]
            n118 = call <vilib>:"WSS.Generate.Digital.vi"("LF Wheel Speed Sensor Settings"="Front Passenger WS.Settings") -> ("Bit1"=w173:bool, "Bit0"=w174:bool)  [unwired: 9 in]
            n119 = call <vilib>:"WSS.Generate.Digital.vi"("LF Wheel Speed Sensor Settings"="Rear Driver WS.Settings") -> ("Bit1"=w170:bool, "Bit0"=w171:bool)  [unwired: 9 in]
            n120 = call <vilib>:"WSS.Generate.Digital.vi"("LF Wheel Speed Sensor Settings"="Read Passenger WS.Settings") -> ("Bit1"=w167:bool, "Bit0"=w168:bool)  [unwired: 9 in]
            n121 = Index Array(array=w159) -> (element #1=→"Relay State":bool, element #2=→"Switch State":bool, element #3=→"Key State":bool, element #4=w154:bool, element #5=w151:bool, element #6=w148:bool, element #7=w136:bool, element #8=w124:bool)  [unwired: 8 in]
            n122 = Build Array(w188, w187, w186, w185, "Key", "Switch", w182, w181) -> (w179:bool[])
            "Connector0 DIO Bank0.Monitor" <- w179
            n123 = call <vilib>:"PWM.Measure.Digital.vi"("State"=w154, "Settings"="PWM IN 1.Settings") -> ("Measurement"=→"PWM IN 1.Measure":T4)  [unwired: 8 in, 1 out]
            n124 = call <vilib>:"PWM.Measure.Digital.vi"("State"=w151, "Settings"="PWM IN 2.Settings") -> ("Measurement"=→"PWM IN 2.Measure":T4)  [unwired: 8 in, 1 out]
            n125 = call-poly <vilib>:"Measure Events.vi"("settings.<user name>"="settings.Cyl Inj 1", "register bus"=w198, "event"=w148) -> ("measured data"=w145:T41, "status.<user name>"=→"status.Cyl Inj 1":T2)  [unwired: 7 in]
            n126 = call-poly <vilib>:"Measure Events.vi"("settings.<user name>"="settings.Cyl Inj 2", "register bus"=w198, "event"=w136) -> ("measured data"=w133:T41, "status.<user name>"=→"status.Cyl Inj 2":T2)  [unwired: 7 in]
            n127 = call-poly <vilib>:"Measure Events.vi"("settings.<user name>"="settings.Cyl Inj 3", "register bus"=w198, "event"=w124) -> ("measured data"=w121:T41, "status.<user name>"=→"status.Cyl Inj 3":T2)  [unwired: 7 in]
            n128 = Build Array(w177, w176) -> (w166:bool[])
            n129 = Build Array(w174, w173) -> (w165:bool[])
            n130 = Build Array(w171, w170) -> (w164:bool[])
            n131 = Build Array(w168, w167) -> (w163:bool[])
            n132 = call "Digital_Output_8Channels.vi"("States"=w179, "IO"=T34 {"DO 0"="Connector0/DIO0", "DO 1"="Connector0/DIO1", "DO 2"="Connector0/DIO2", "DO 3"="Connector0/DIO3", "DO 4"="Connector0/DIO4", "DO 5"="Connector0/DIO5", "DO 6"="Connector0/DIO6", "DO 7"="Connector0/DIO7"}) -> ()  [unwired: 1 in]
            n133 = Build Array (concatenate)(w166, w165, w164, w163) -> (w161:bool[])
            "Connector0 DIO Bank1.Monitor" <- w161
            n134 = call <vilib>:"Capture Event.vi"("event # to capture"=T32 1, "measured data"=w145) -> ("capture.<user name>"=→"capture.Cyl Inj 1.Event 1":T1)  [unwired: 9 in]
            n135 = call <vilib>:"Capture Event.vi"("event # to capture"=T32 2, "measured data"=w145) -> ("capture.<user name>"=→"capture.Cyl Inj 1.Event 2":T1)  [unwired: 9 in]
            n136 = call <vilib>:"Capture Event.vi"("event # to capture"=T32 3, "measured data"=w145) -> ("capture.<user name>"=→"capture.Cyl Inj 1.Event 3":T1)  [unwired: 9 in]
            n137 = call <vilib>:"Capture Event.vi"("event # to capture"=T32 4, "measured data"=w145) -> ("capture.<user name>"=→"capture.Cyl Inj 1.Event 4":T1)  [unwired: 9 in]
            n138 = call <vilib>:"Capture Event.vi"("event # to capture"=T32 1, "measured data"=w133) -> ("capture.<user name>"=→"capture.Cyl Inj 2.Event 1":T1)  [unwired: 9 in]
            n139 = call <vilib>:"Capture Event.vi"("event # to capture"=T32 2, "measured data"=w133) -> ("capture.<user name>"=→"capture.Cyl Inj 2.Event 2":T1)  [unwired: 9 in]
            n140 = call <vilib>:"Capture Event.vi"("event # to capture"=T32 3, "measured data"=w133) -> ("capture.<user name>"=→"capture.Cyl Inj 2.Event 3":T1)  [unwired: 9 in]
            n141 = call <vilib>:"Capture Event.vi"("event # to capture"=T32 4, "measured data"=w133) -> ("capture.<user name>"=→"capture.Cyl Inj 2.Event 4":T1)  [unwired: 9 in]
            n142 = call <vilib>:"Capture Event.vi"("event # to capture"=T32 1, "measured data"=w121) -> ("capture.<user name>"=→"capture.Cyl Inj 3.Event 1":T1)  [unwired: 9 in]
            n143 = call <vilib>:"Capture Event.vi"("event # to capture"=T32 2, "measured data"=w121) -> ("capture.<user name>"=→"capture.Cyl Inj 3.Event 2":T1)  [unwired: 9 in]
            n144 = call <vilib>:"Capture Event.vi"("event # to capture"=T32 3, "measured data"=w121) -> ("capture.<user name>"=→"capture.Cyl Inj 3.Event 3":T1)  [unwired: 9 in]
            n145 = call <vilib>:"Capture Event.vi"("event # to capture"=T32 4, "measured data"=w121) -> ("capture.<user name>"=→"capture.Cyl Inj 3.Event 4":T1)  [unwired: 9 in]
            n146 = call "Digital_Output_8Channels.vi"("States"=w161, "IO"=T34 {"DO 0"="Connector0/DIO8", "DO 1"="Connector0/DIO9", "DO 2"="Connector0/DIO10", "DO 3"="Connector0/DIO11", "DO 4"="Connector0/DIO12", "DO 5"="Connector0/DIO13", "DO 6"="Connector0/DIO14", "DO 7"="Connector0/DIO15"}) -> ()  [unwired: 1 in]
          }
        }
      }
      n147 = node-c288 ("Output Node")(w97) -> ()
      n148 = node-c288 ("Output Node")(w99) -> ()
    }
  }
